vi "Review Fiducials.vi"(7 "Console Log in":refnum<class "Console Log.lvclass">, 8 "error in":errorcluster, 11 "Gluing Procedure in":refnum<class "Gluing Procedure.lvclass">) -> (0 "error out":errorcluster, 1 "Step canceled?":bool, 3 "Gluing Procedure out":refnum<class "Gluing Procedure.lvclass">, 5 "Console Log out":refnum<class "Console Log.lvclass">)   [LabVIEW 2011]
uses:
  Procedure Classes/Gluing Procedure/Gluing Procedure.lvclass
  Application Utilities/Console Log/Console Log.lvclass
  Shared Components/WorkTable Class/Type Definitions/Worktable_Mode.ctl
  Shared Components/Utils/Type Definitions/Fiducial with Source.ctl
  Shared Components/Vec3d Class/Vec3d Class.lvclass
  Procedure Classes/Gluing Procedure/Type Definitions/Review Fuducials.ctl
  Procedure Classes/Gluing Procedure/Type Definitions/Inspect Fuducials.ctl
  Shared Components/Utils/Type Definitions/Part Fiducials.ctl
  Shared Components/Utils/Type Definitions/Fiducial Image.ctl
  Shared Components/Utils/Type Definitions/Physical Image.ctl
  <vilib>/vision/Image Controls.llb/IMAQ Image.ctl
panel:
  in  "idx value":i32
  out "idx_label":string="1/10"
  in  "Previous":bool
  in  "Next":bool
  in  "Path Tab Control":T1(tab)
  out "BBM Slot":i32
  in  "reacquire BBM BL":bool
  in  "reacquire BBM BR":bool
  in  "reacquire BBM TR":bool
  out "BBM TR View":T2(plugin-control)
  out "BBM TL View":T2(plugin-control)
  out "BBM BR View":T2(plugin-control)
  out "BBM BL View":T2(plugin-control)
  in  "reacquire BBM TL":bool
  in  "reacquire HDI TL":bool
  out "HDI BL View":T2(plugin-control)
  out "HDI BR View":T2(plugin-control)
  out "HDI TL View":T2(plugin-control)
  out "HDI TR View":T2(plugin-control)
  in  "reacquire HDI TR":bool
  in  "reacquire HDI BR":bool
  in  "reacquire HDI BL":bool
  out "HDI Slot":i32
  in  "reacquire Stamp BL":bool
  in  "reacquire Stamp BR":bool
  in  "reacquire Stamp TR":bool
  out "Stamp TR View":T2(plugin-control)
  out "Stamp TL View":T2(plugin-control)
  out "Stamp BR View":T2(plugin-control)
  out "Stamp BL View":T2(plugin-control)
  in  "reacquire Stamp TL":bool
  out "Stamp Slot":i32
  in  "reacquire Weight TL":bool
  out "Weight BL View":T2(plugin-control)
  out "Weight BR View":T2(plugin-control)
  out "Weight TL View":T2(plugin-control)
  out "Weight TR View":T2(plugin-control)
  in  "reacquire Weight TR":bool
  in  "reacquire Weight BR":bool
  in  "reacquire Weight BL":bool
  out "Weight Slot":i32
  in  "Cancel Button":bool
  in  "OK Button":bool
  # "This is going to be a monstrous VI.\n\nThis VI needs to display the fiducial images to the user for all HDI, Stamps, Weights, and BBMs.  Users can accept camera's findings or user designate fiducial centers.\n\nHitting okay will write fidicial coords to worktable."
  # "Click on images to correct fiducial positions.\nAll error fiducials must be corrected before continuing."
  # "Pattern Recognition"
  # "Error"
  # "User Defined"
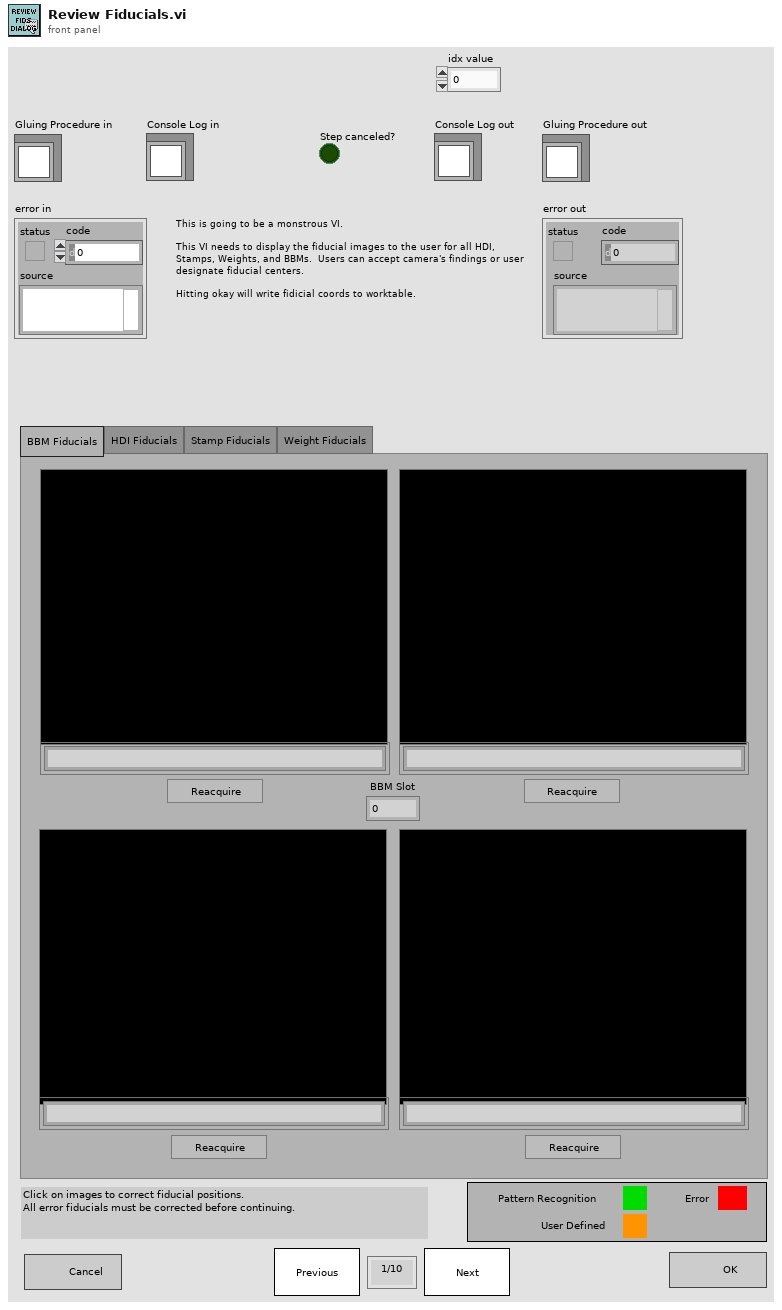
[diagram p1: front panel]
types:
  T1 = enum32{"BBM Fiducials", "HDI Fiducials", "Stamp Fiducials", "Weight Fiducials"}
  T2 = typedef "IMAQ Image.ctl" = refnum<image>
  T3 = cluster{"reacq. HDI":refnum<vi>[], "reacq. Stamp":refnum<vi>[], "reacq. Weight":refnum<vi>[], "reacq. BBM":refnum<vi>[]}
  T4 = typedef "Inspect Fuducials.ctl" = cluster{"Path Fiducials":cluster{"HDI Fiducials":T5, "Stamp Fiducials":T5, "Weight Fiducials":T5, "BBM Fiducials":T5}[], "Has been run?":bool}
  T5 = typedef "Part Fiducials.ctl" = cluster{"Fiducials":T6[], "Chuck":i32, "Slot":i32}
  T6 = typedef "Fiducial Image.ctl" = cluster{"Fiducial Image":T7, "Selected Fiducial":T8, "fiducial name":string}
  T7 = typedef "Physical Image.ctl" = cluster{"Image Position":refnum<class "Vec3d Class.lvclass">, "Image Reference":T2, "Field of View":cluster{"x(mm)":dbl, "y(mm)":dbl}}
  T8 = typedef "Fiducial with Source.ctl" = cluster{"Fiducial Image Coordinate":refnum<class "Vec3d Class.lvclass">, "Fiducial Source":enum16{"Pattern Recognition", "User", "Error", "Default"}}
  T9 = cluster{"HDI Fiducials":T5, "Stamp Fiducials":T5, "Weight Fiducials":T5, "BBM Fiducials":T5}[]
  T10 = typedef "Worktable_Mode.ctl" = enum16{"Encapsulation", "Gluing"}
  T11 = enum16{"None", "glue_resevoir_chuck", "stamp_tool_chuck", "weight_tool_chuck", "hdi_chuck_04"}
  T12 = enum16{"None", "glue_resevoir_chuck", "stamp_tool_chuck", "weight_tool_chuck"}
  T13 = enum16{"Pattern Recognition", "User", "Error", "Default"}
  T14 = typedef "eventvkey.ctl" = enum16{"ASCII", "Enter", "Return", "Shift", "Ctrl", "Alt", "Cmd", "Opt", "Caps", "NumLock", "Clear", "Break", "Up", "Down", "Left", "Right", "Insert", "Delete", "Home", "End", "PageUp", "PageDown", "Escape", "Help", "Pause", "ScrollLock", "F1", "F2", "F3", "F4", "F5", "F6", "F7", "F8", "F9", "F10", "F11", "F12", "F13", "F14", "F15", "F16", "F17", "F18", "F19", "F20", "F21", "F22", "F23", "F24", "Play", "VolumeUp", "VolumeDown", "Mute", "Two Byte Char"}
  T15 = cluster{"HDI Fiducials":T5, "Stamp Fiducials":T5, "Weight Fiducials":T5, "BBM Fiducials":T5}
  T16 = typedef "LVPoint32TypeDef.ctl" = cluster{"Horizontal":i32, "Vertical":i32}
  T17 = typedef "Review Fuducials.ctl" = cluster{"Has been run?":bool}
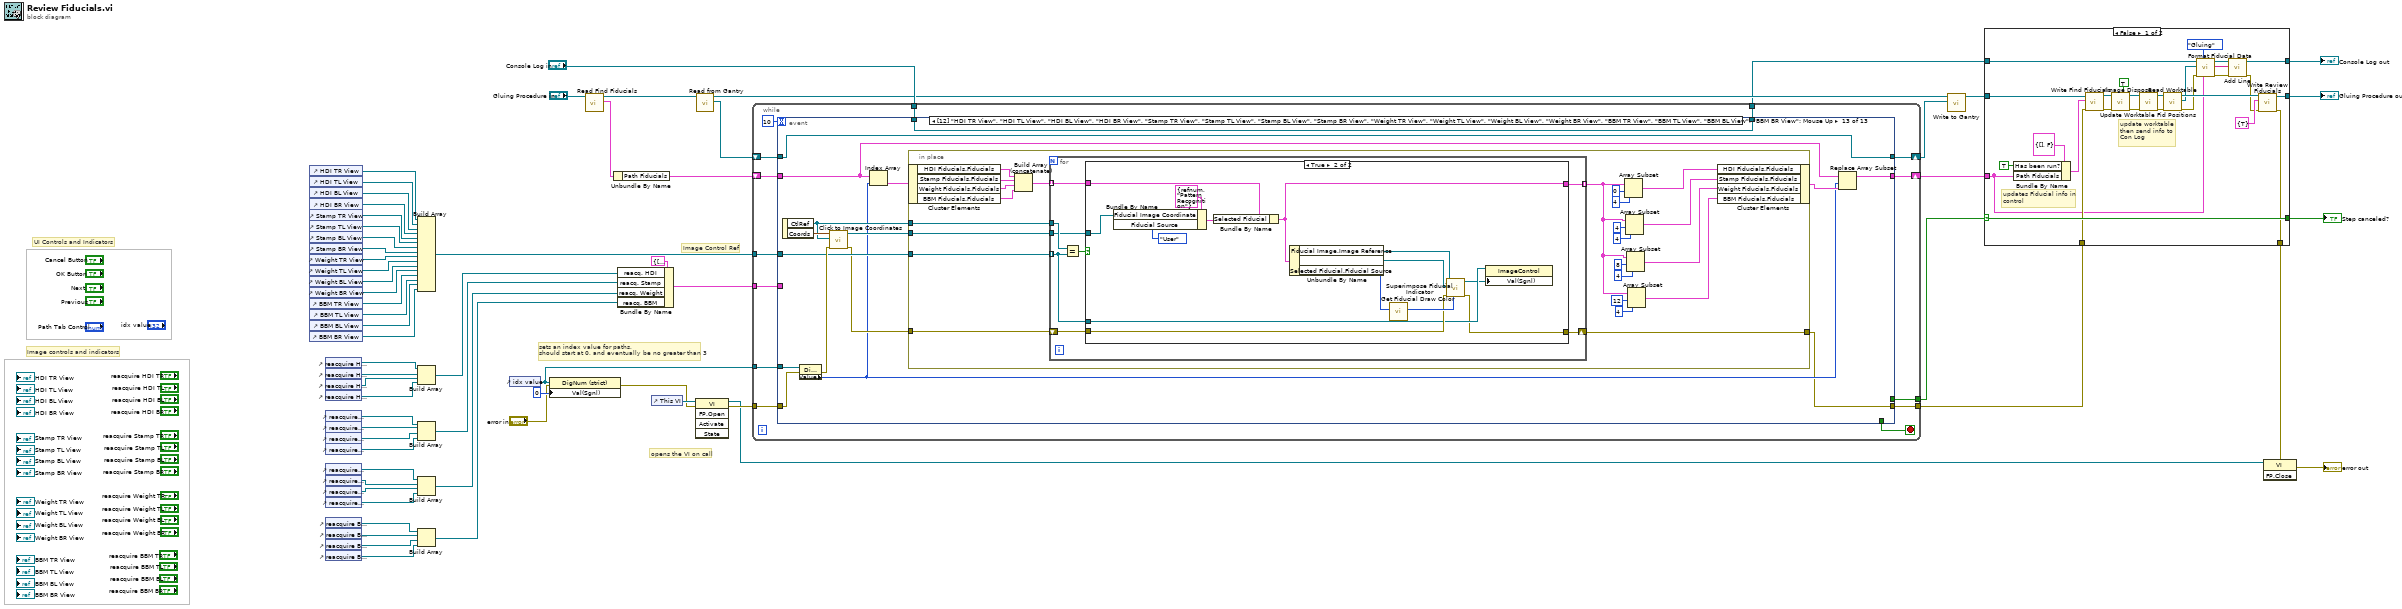
[diagram p0: block diagram]
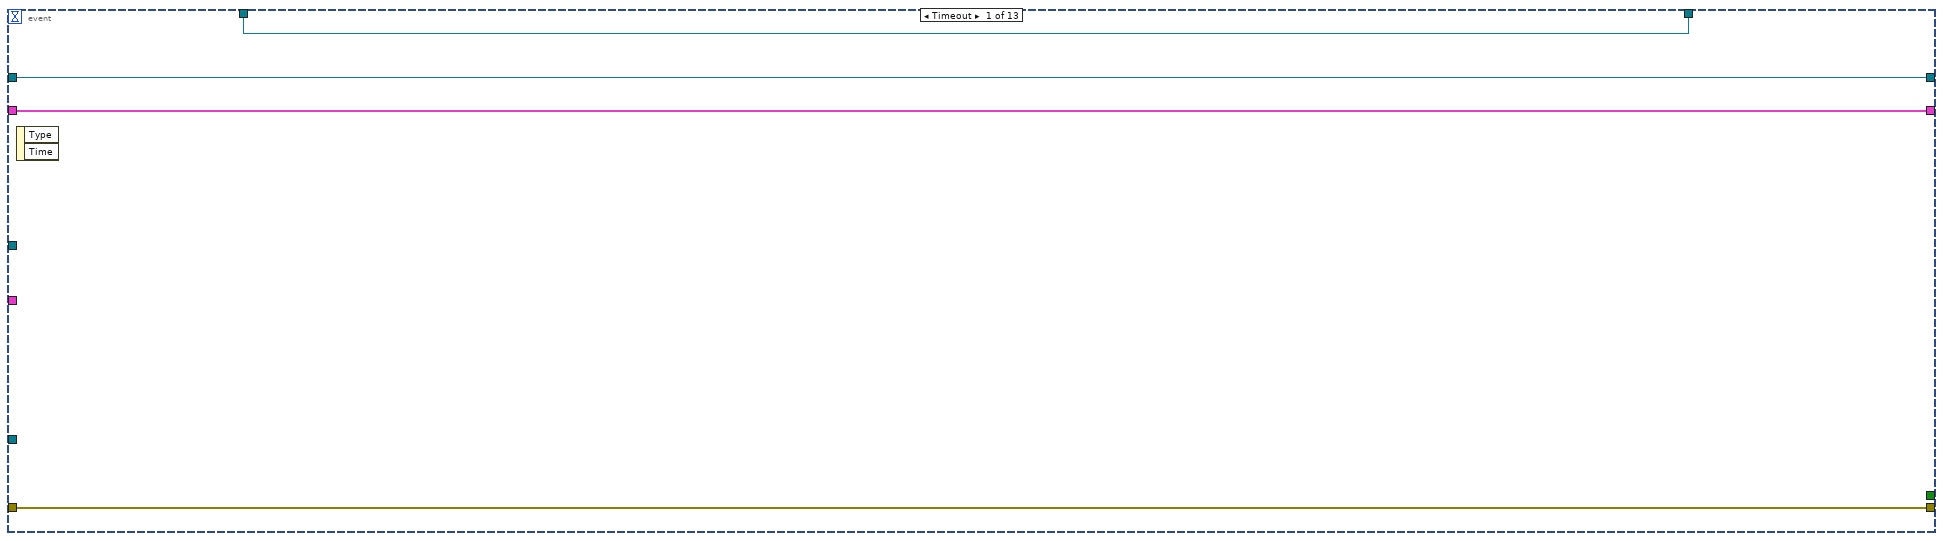
[diagram p3: hidden frame]
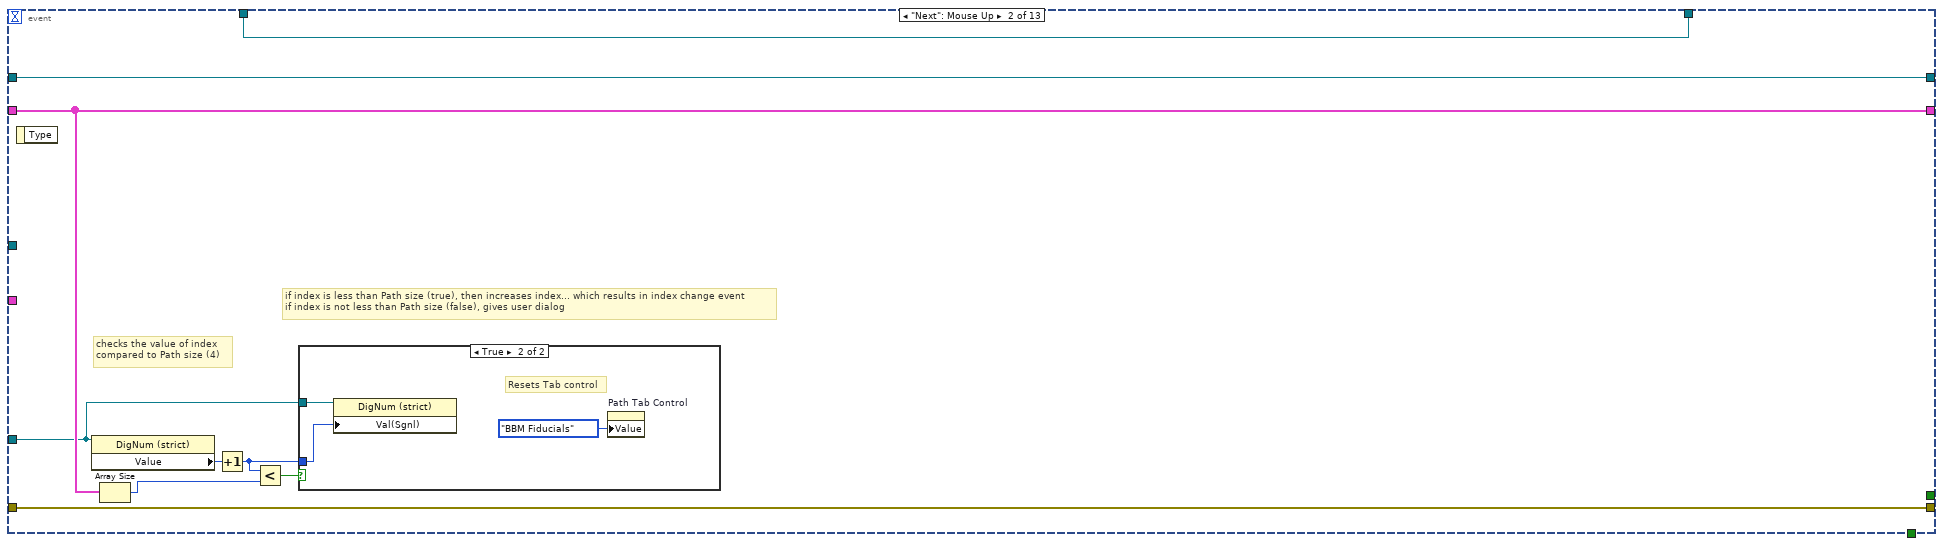
[diagram p4: hidden frame]
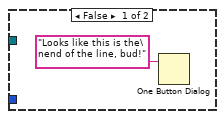
[diagram p5: hidden frame]
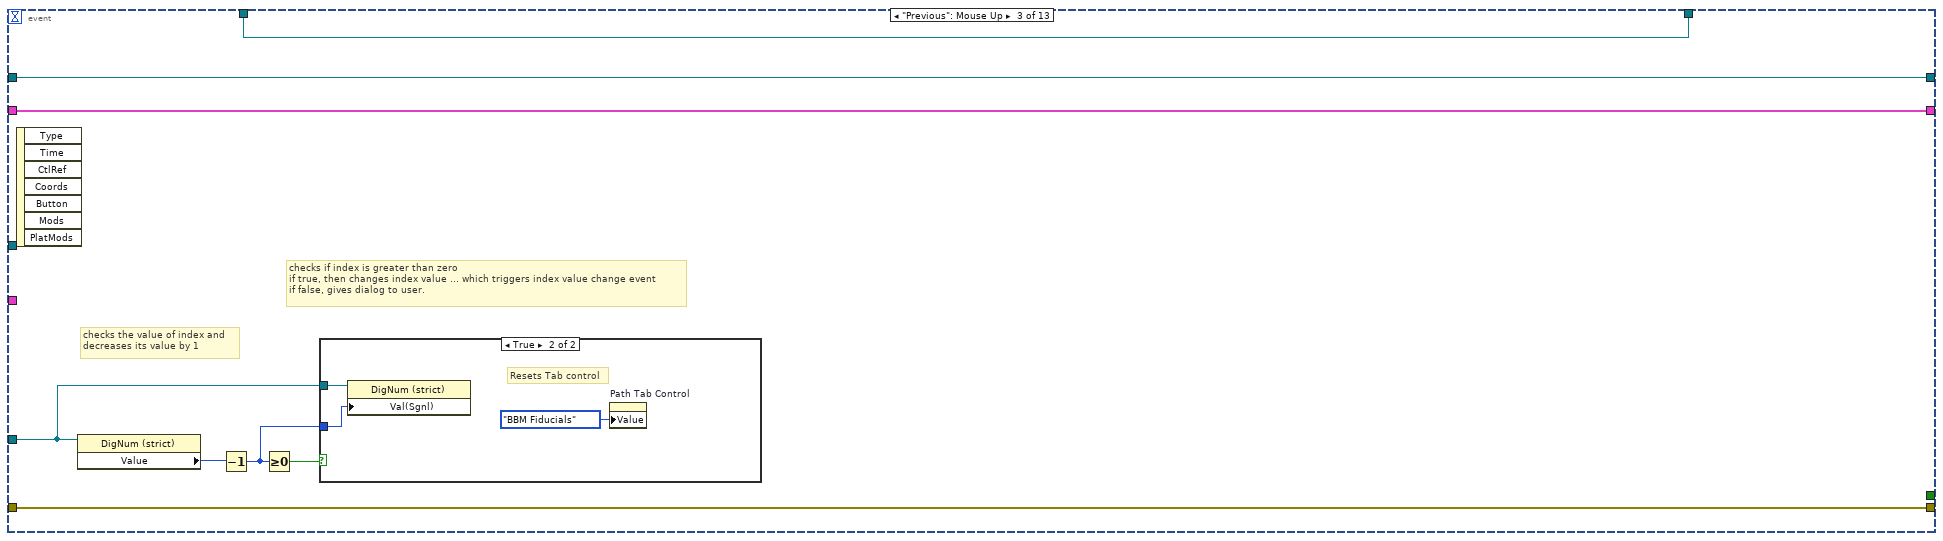
[diagram p6: hidden frame]
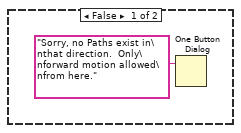
[diagram p7: hidden frame]
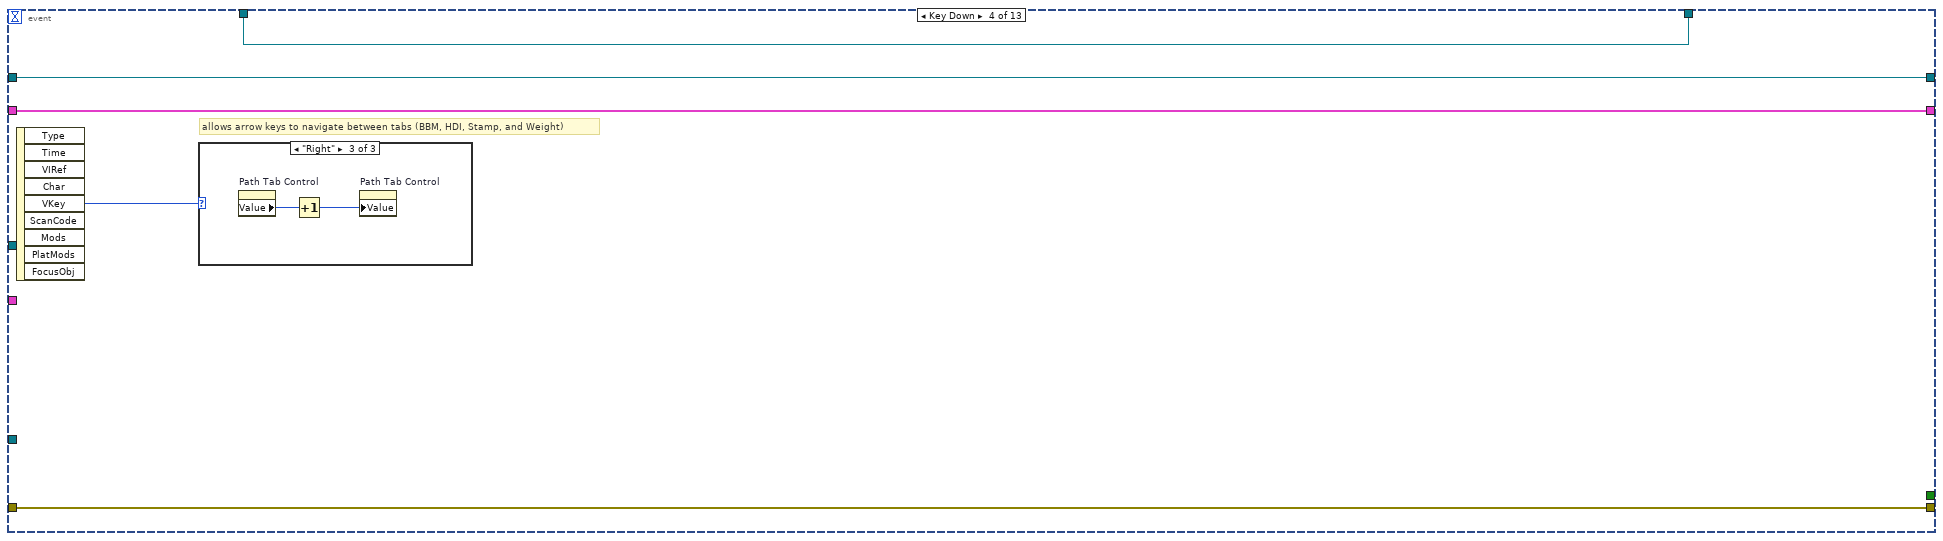
[diagram p8: hidden frame]
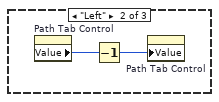
[diagram p10: hidden frame]
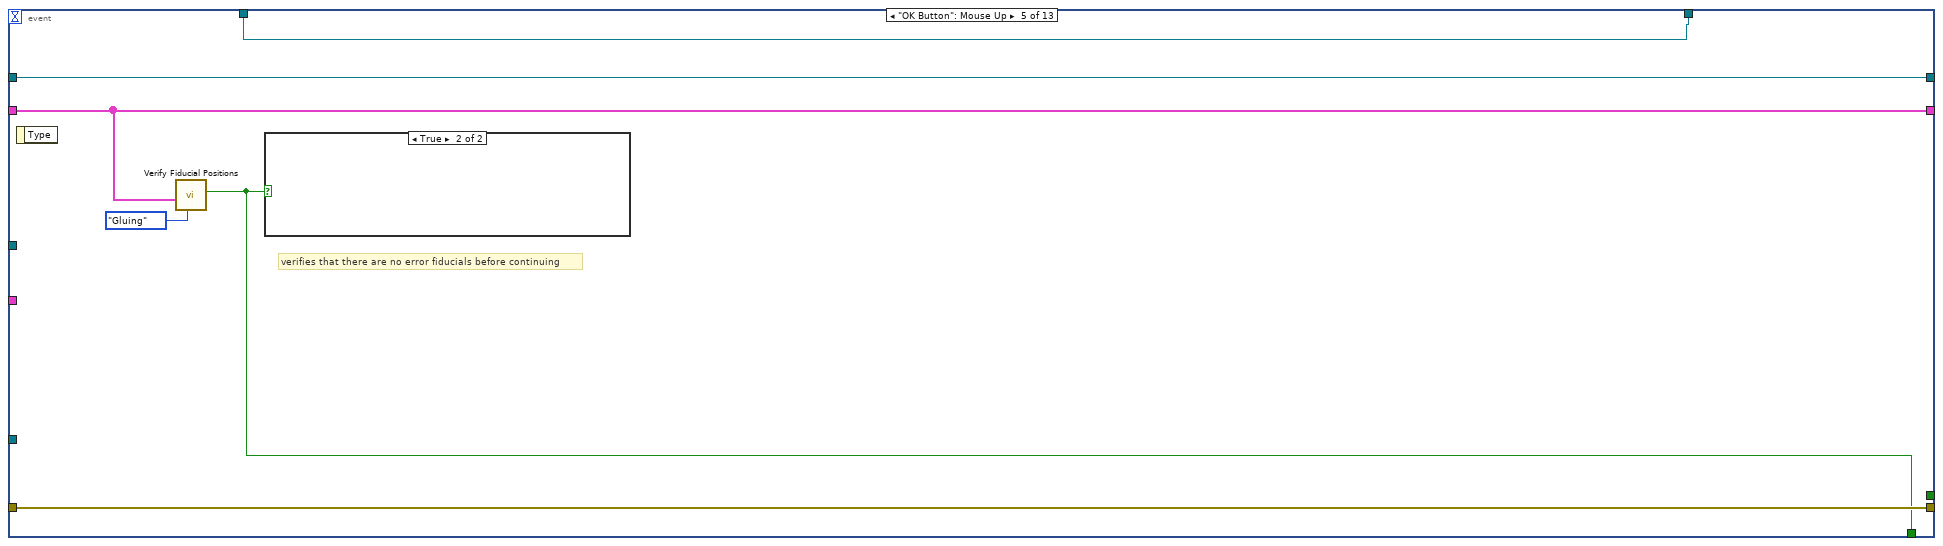
[diagram p11: hidden frame]
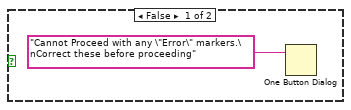
[diagram p12: hidden frame]
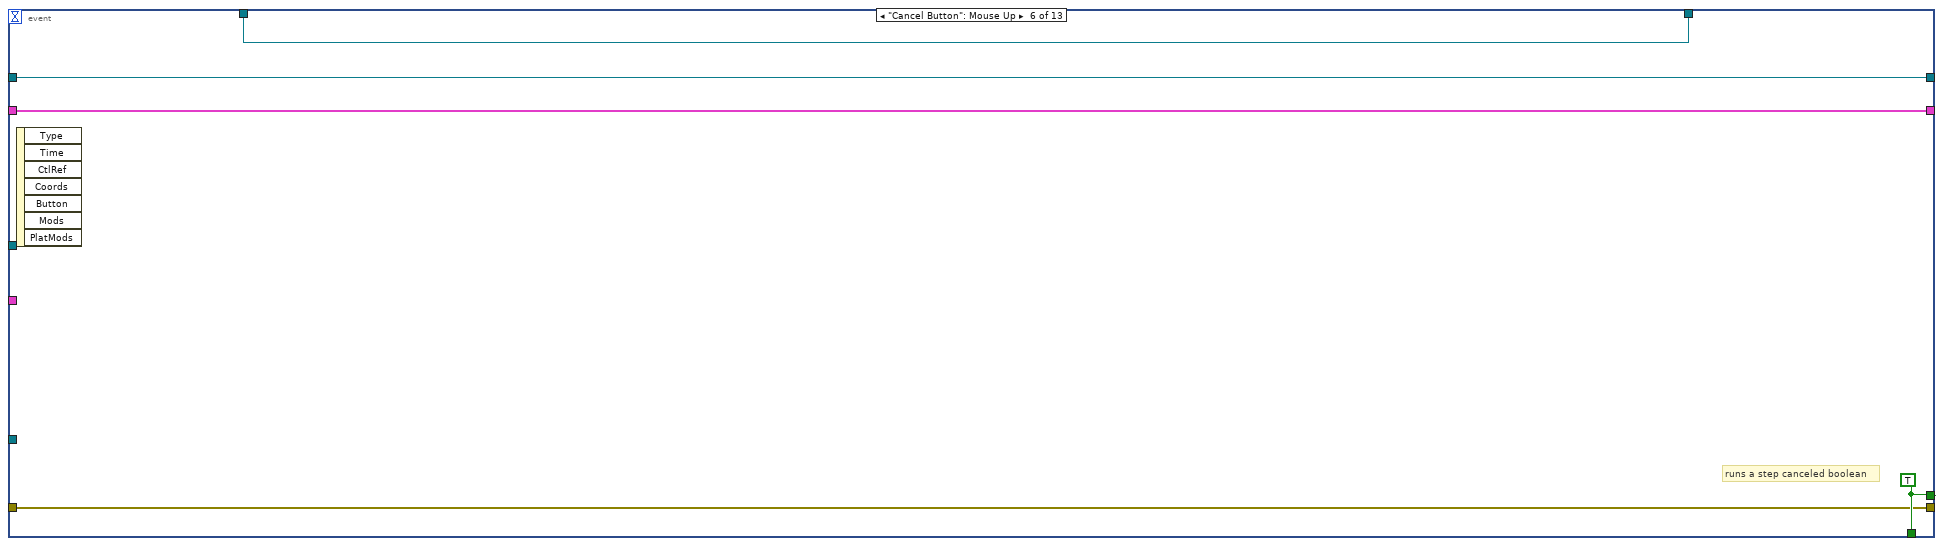
[diagram p13: hidden frame]
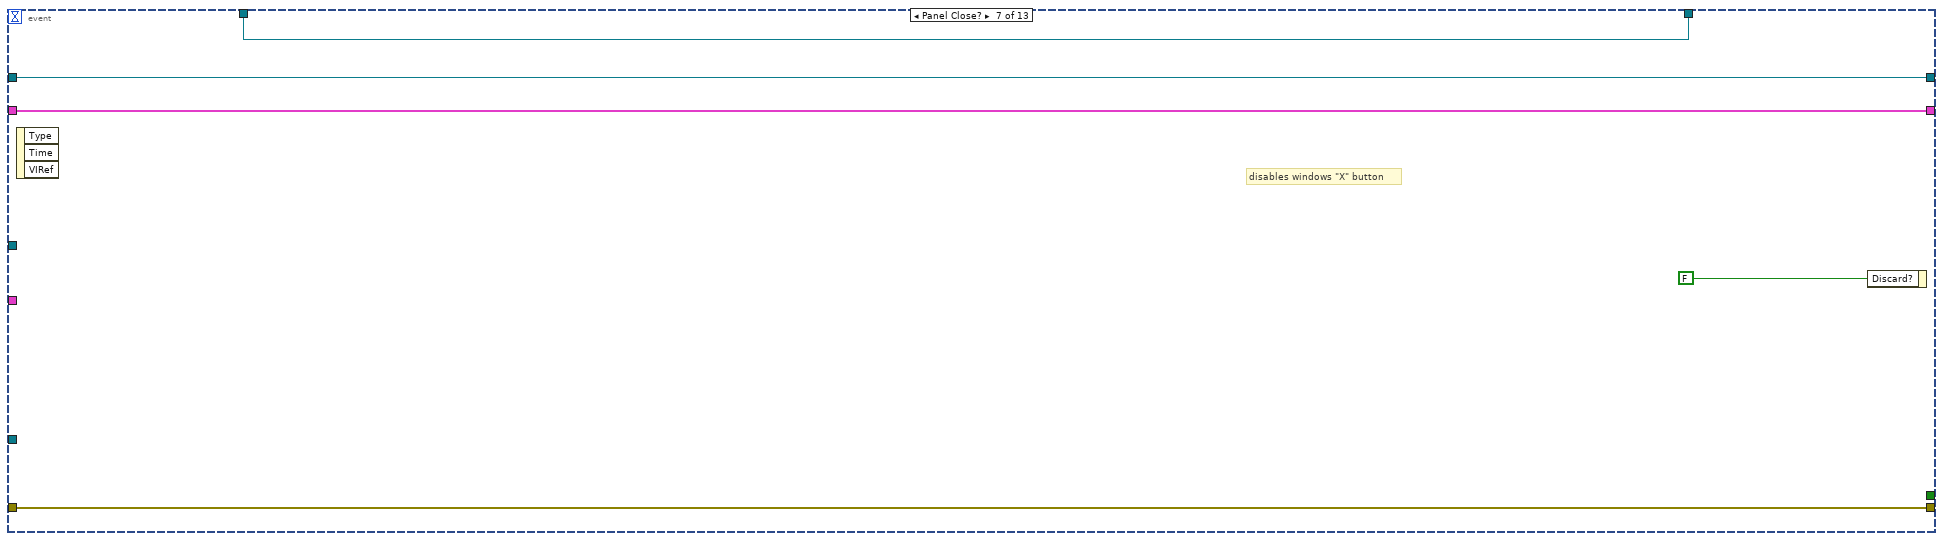
[diagram p14: hidden frame]
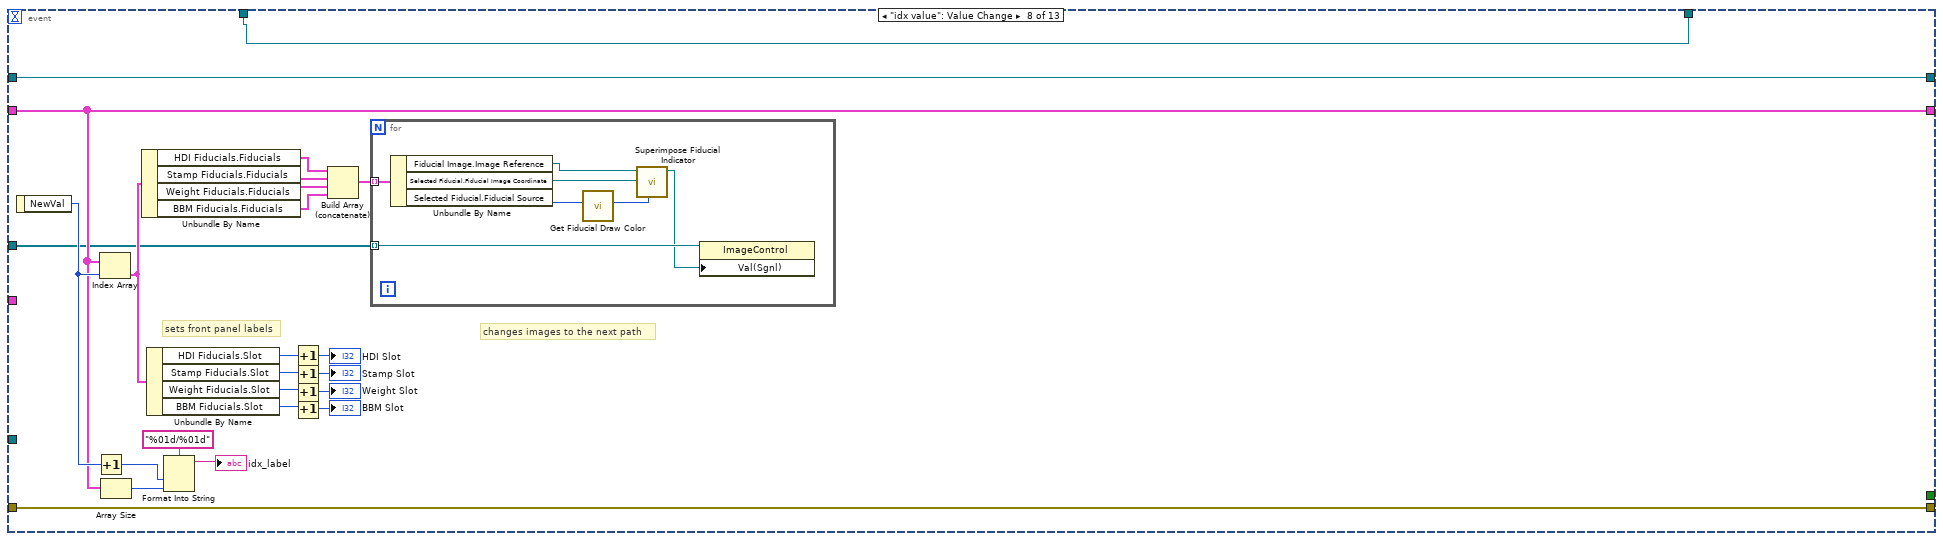
[diagram p15: hidden frame]
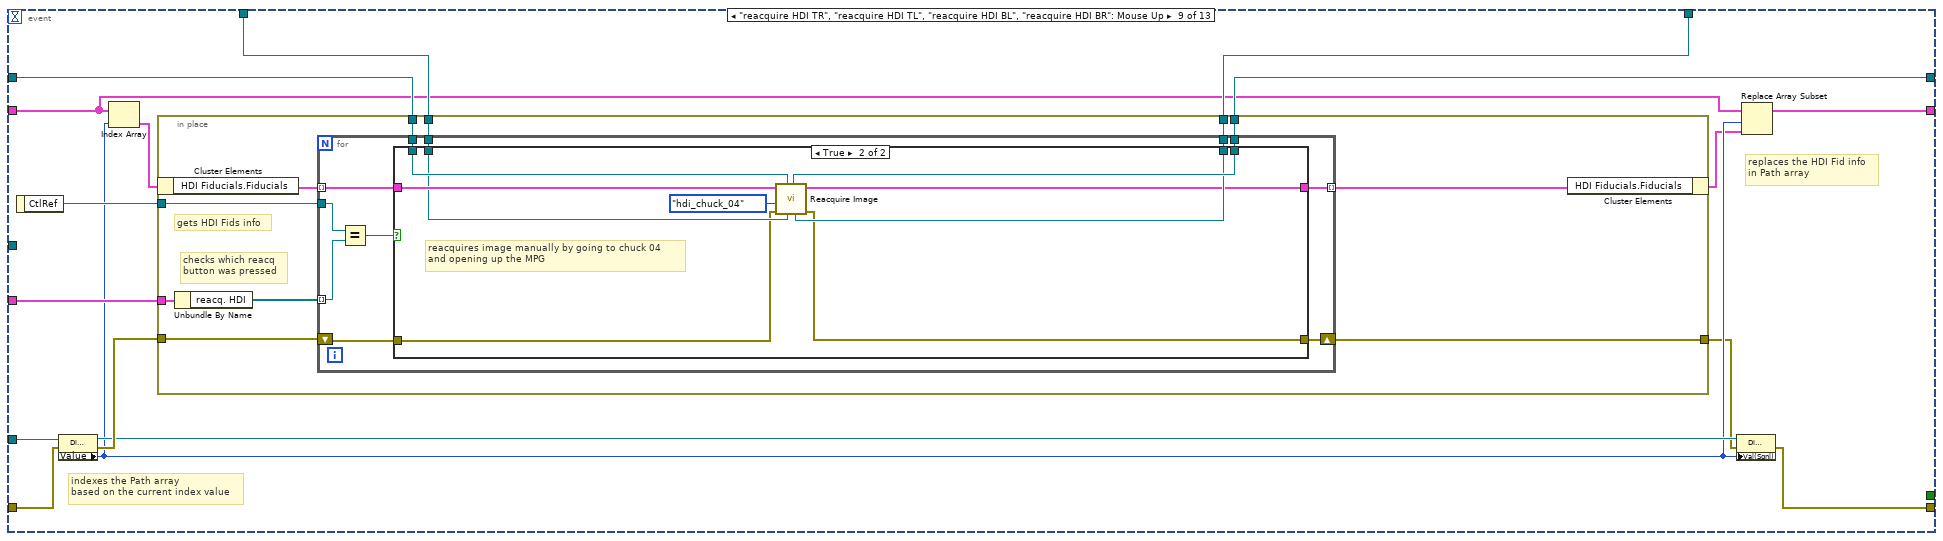
[diagram p16: hidden frame]
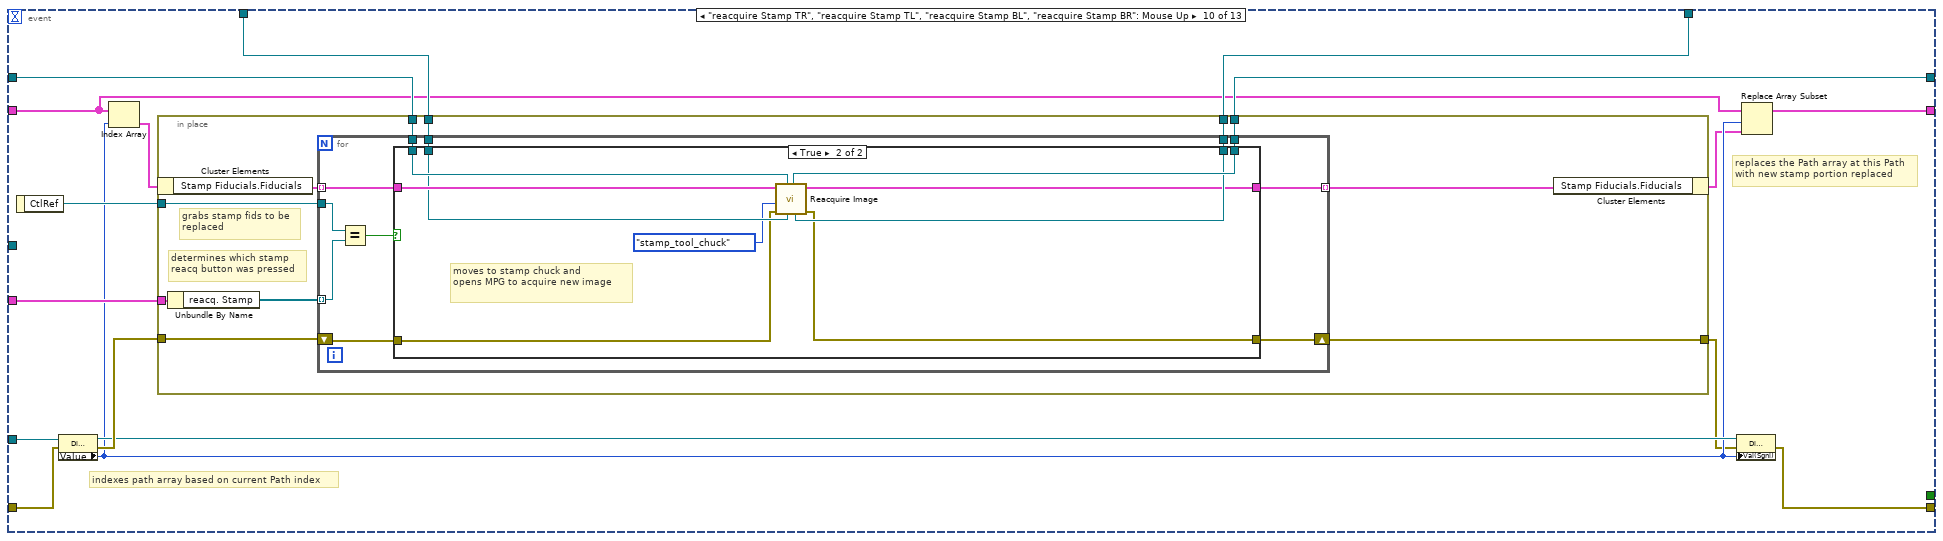
[diagram p18: hidden frame]
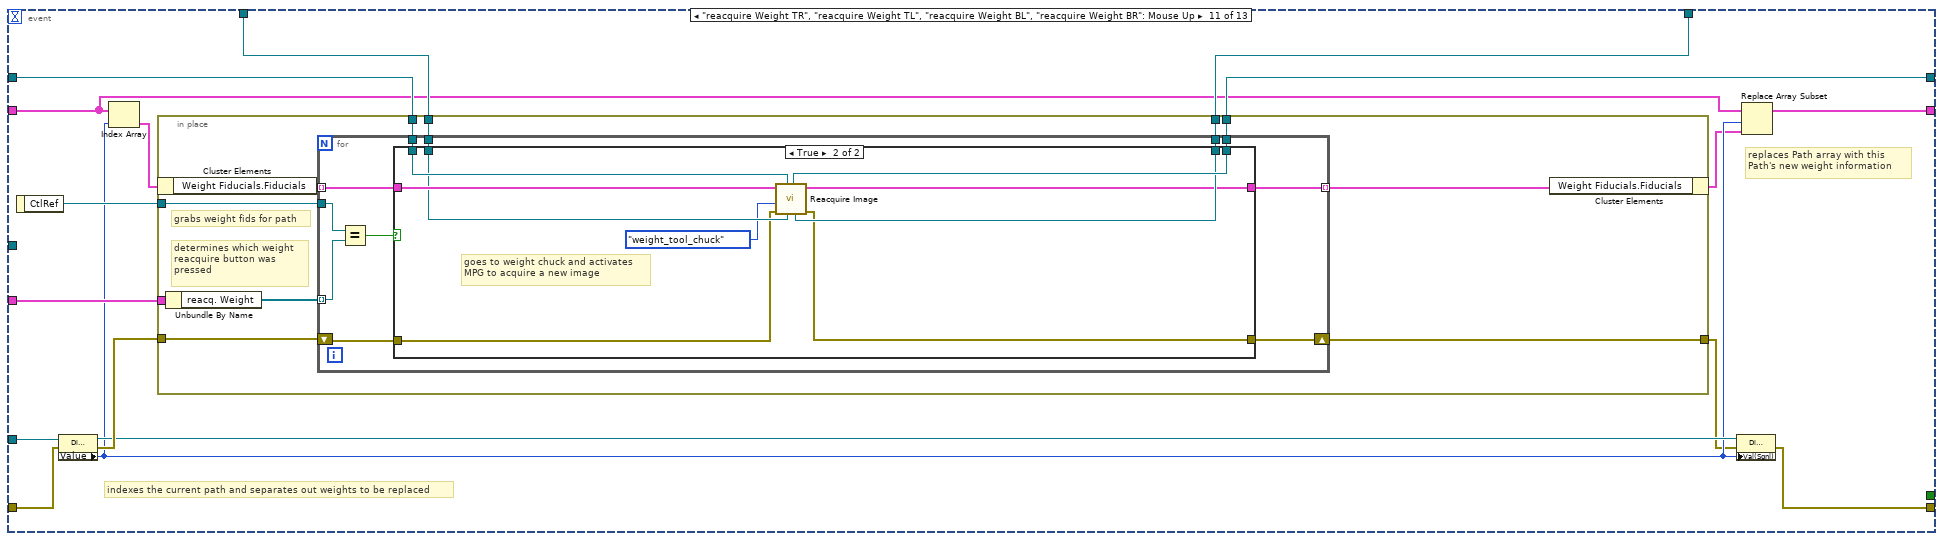
[diagram p20: hidden frame]
diagram:
  # "opens the VI on call"
  # "sets an index value for paths,\nshould start at 0, and eventually be no greater than 3"
  # "Image controls and indicators"
  # "UI Controls and Indicators"
  # "Image Control Ref"
  n1 = control-ref of="HDI TR View"() -> (w54:refnum<vi>)
  n2 = control-ref of="HDI TL View"() -> (w53:refnum<vi>)
  n3 = control-ref of="HDI BL View"() -> (w52:refnum<vi>)
  n4 = control-ref of="HDI BR View"() -> (w51:refnum<vi>)
  n5 = control-ref of="Stamp TR View"() -> (w50:refnum<vi>)
  n6 = control-ref of="Stamp TL View"() -> (w49:refnum<vi>)
  n7 = control-ref of="Stamp BL View"() -> (w48:refnum<vi>)
  n8 = control-ref of="Stamp BR View"() -> (w47:refnum<vi>)
  n9 = control-ref of="Weight TR View"() -> (w46:refnum<vi>)
  n10 = control-ref of="Weight TL View"() -> (w45:refnum<vi>)
  n11 = control-ref of="Weight BL View"() -> (w44:refnum<vi>)
  n12 = control-ref of="Weight BR View"() -> (w43:refnum<vi>)
  n13 = control-ref of="BBM TR View"() -> (w42:refnum<vi>)
  n14 = control-ref of="BBM TL View"() -> (w41:refnum<vi>)
  n15 = control-ref of="BBM BL View"() -> (w40:refnum<vi>)
  n16 = control-ref of="BBM BR View"() -> (w39:refnum<vi>)
  n17 = control-ref of="reacquire HDI TR"() -> (w37:refnum<vi>)
  n18 = control-ref of="reacquire HDI TL"() -> (w36:refnum<vi>)
  n19 = control-ref of="reacquire HDI BL"() -> (w35:refnum<vi>)
  n20 = control-ref of="reacquire HDI BR"() -> (w34:refnum<vi>)
  n21 = control-ref of="reacquire Stamp TR"() -> (w33:refnum<vi>)
  n22 = control-ref of="reacquire Stamp TL"() -> (w32:refnum<vi>)
  n23 = control-ref of="reacquire Stamp BL"() -> (w31:refnum<vi>)
  n24 = control-ref of="reacquire Stamp BR"() -> (w30:refnum<vi>)
  n25 = control-ref of="reacquire Weight TR"() -> (w29:refnum<vi>)
  n26 = control-ref of="reacquire Weight TL"() -> (w28:refnum<vi>)
  n27 = control-ref of="reacquire Weight BL"() -> (w27:refnum<vi>)
  n28 = control-ref of="reacquire Weight BR"() -> (w26:refnum<vi>)
  n29 = control-ref of="reacquire BBM TR"() -> (w25:refnum<vi>)
  n30 = control-ref of="reacquire BBM TL"() -> (w24:refnum<vi>)
  n31 = control-ref of="reacquire BBM BL"() -> (w23:refnum<vi>)
  n32 = control-ref of="reacquire BBM BR"() -> (w22:refnum<vi>)
  n33 = Build Array(w54, w53, w52, w51, w50, w49, w48, w47, w46, w45, w44, w43, w42, w41, w40, w39) -> (w38:refnum<vi>[])
  n34 = Build Array(w37, w36, w35, w34) -> (w20:refnum<vi>[])
  n35 = Build Array(w33, w32, w31, w30) -> (w18:refnum<vi>[])
  n36 = Build Array(w29, w28, w27, w26) -> (w17:refnum<vi>[])
  n37 = Build Array(w25, w24, w23, w22) -> (w16:refnum<vi>[])
  n38 = control-ref of="idx value"() -> (w55:refnum<vi>)
  n39 = property class="DigNum (strict)"(reference=w55, error in="error in", "Val(Sgnl)"=0 ("Value (Signaling)")) -> (error out=w56:errorcluster)  [unwired: 1 out]
  n40 = call "Read Find Fiducials.vi"("Gluing Procedure in"="Gluing Procedure in") -> ("Find Fiducials"=w62:T4, "Gluing Procedure out"=w61:refnum<class "Gluing Procedure.lvclass">)  [unwired: 8 in, 1 out]
  n41 = Unbundle By Name(w62) -> ("Path Fiducials"=w1:T9)
  n42 = Bundle By Name(cluster=T3 {"reacq. HDI"=[], "reacq. Stamp"=[], "reacq. Weight"=[], "reacq. BBM"=[]}, "reacq. HDI"=w20, "reacq. Stamp"=w18, "reacq. Weight"=w17, "reacq. BBM"=w16) -> (w19:T3)
  n43 = control-ref of="This VI"() -> (w64:refnum<vi>)
  n44 = invoke class="VI" method="FP.Open"(reference=w64, error in=w56) -> (reference out=w15:refnum<vi>, error out=w59:errorcluster)  [unwired: 3 in, 3 out]
  n45 = call "Read from Gantry.vi"("Gluing Procedure in"=w61) -> ("Gantry"=w60:refnum<class "Gantry Class.lvclass">, "Gluing Procedure out"=w14:refnum<class "Gluing Procedure.lvclass">)  [unwired: 8 in, 1 out]
  n46 = while {
    tunnel: "Console Log in" -> [w73]
    shift-right: [w75] -> w13
    shift-left: w60 -> [w76]
    shift-right: [w74] -> w9
    shift-left: w1 -> [w77]
    tunnel: [w72] -> w8
    tunnel: w59 -> [w71]
    tunnel: [w70] -> w5
    tunnel: [w68] -> w11
    tunnel: w55 -> [w67]
    tunnel: w38 -> [w66]
    tunnel: w19 -> [w65]
    stop <- w69 stop-if-true
    n47 = event shown="[12] \"HDI TR View\", \"HDI TL View\", \"HDI BL View\", \"HDI BR View\", \"Stamp TR View\", \"Stamp TL View\", \"Stamp BL View\", \"Stamp BR View\", \"Weight TR View\", \"Weight TL View\", \"Weight BL View\", \"Weight BR View\", \"BBM TR View\", \"BBM TL View\", \"BBM BL View\", \"BBM BR View\": Mouse Up" {
      selector: _ -> [_ _ _ _ _ _ _ _ _ _ _ _ _]
      dyn-events: _ -> [_ _ _ _ _ _ _ _ _ _ _ _ _]
      timeout: 10 -> [_ _ _ _ _ _ _ _ _ _ _ _ _]
      tunnel: w77 -> [w81 w89 w102 w110 w120 w127 w131 w154 w170 w222 w274 w326 w383]
      tunnel: w76 -> [w82 w91 w103 w111 w121 w128 w132 w157 w177 w229 w281 w333 w380]
      tunnel: [w82 w91 w103 w111 w121 w128 w132 w157 w176 w228 w280 w332 w380] -> w75
      tunnel: [w81 w89 w102 w110 w120 w127 w131 w154 w167 w219 w271 w323 w381] -> w74
      tunnel: w73 -> [w80 w83 w96 w109 w118 w124 w129 w142 w175 w227 w279 w331 w378]
      tunnel: [w80 w83 w96 w109 w118 w124 w129 w142 w174 w226 w278 w330 w378] -> w72
      tunnel: w71 -> [w79 w90 w101 w108 w122 w125 w130 w156 w180 w232 w284 w336 w391]
      tunnel: [w79 w90 w101 w108 w122 w125 w130 w156 w165 w217 w269 w321 w379] -> w70
      tunnel: [_ _ _ _ w119 w126 _ _ _ _ _ _ _] -> w69
      tunnel: [_ _ _ _ _ w126 _ _ _ _ _ _ _] -> w68
      tunnel: w67 -> [_ w85 w97 _ _ _ _ _ w181 w233 w285 w337 w392]
      tunnel: w66 -> [_ _ _ _ _ _ _ w143 _ _ _ _ w388]
      tunnel: w65 -> [_ _ _ _ _ _ _ _ w173 w225 w277 w329 _]
      event Timeout {
        n48 = event-data() -> ()  [unwired: 1 in, 2 out]
      }
      event "Next": Mouse Up {
        # "if index is less than Path size (true), then increases index... which results in index change event\nif index is not less than Path size (false), gives user dialog"
        # "checks the value of index \ncompared to Path size (4)"
        n49 = event-data() -> ()  [unwired: 1 in, 1 out]
        n50 = property class="DigNum (strict)"(reference=w85) -> ("Value"=w88:i32)  [unwired: 1 in, 2 out]
        n51 = Array Size(array=w89) -> (size(s)=w87:i32)
        n52 = Increment(x=w88) -> (x+1=w84:i32)
        n53 = Less?(x=w84, y=w87) -> (x < y?=w86:bool)
        n54 = case shown="True" w86 {
          tunnel: w85 -> [_ w95]
          tunnel: w84 -> [_ w94]
          frame False {
            n55 = One Button Dialog(message="Looks like this is the\nend of the line, bud!") -> ()  [unwired: 1 in, 1 out]
          }
          frame True {
            # "Resets Tab control"
            n56 = property class="DigNum (strict)"(reference=w95, "Val(Sgnl)"=w94) -> ()  [unwired: 1 in, 2 out]
            n57 = property on="Path Tab Control" class="TabCtl (strict)"("Value"=T1."BBM Fiducials" ("Path Tab Control")) -> ()  [unwired: 2 in, 2 out]
          }
        }
      }
      event "Previous": Mouse Up {
        # "checks if index is greater than zero\nif true, then changes index value ... which triggers index value change event\nif false, gives dialog to user."
        # "checks the value of index and\ndecreases its value by 1"
        n58 = event-data() -> ()  [unwired: 1 in, 7 out]
        n59 = property class="DigNum (strict)"(reference=w97) -> ("Value"=w100:i32)  [unwired: 1 in, 2 out]
        n60 = Decrement(x=w100) -> (x-1=w98:i32)
        n61 = Greater Or Equal To 0?(x=w98) -> (x >= 0?=w99:bool)
        n62 = case shown="True" w99 {
          tunnel: w98 -> [_ w106]
          tunnel: w97 -> [_ w107]
          frame False {
            n63 = One Button Dialog(message="Sorry, no Paths exist in\nthat direction.  Only\nforward motion allowed\nfrom here.") -> ()  [unwired: 1 in, 1 out]
          }
          frame True {
            # "Resets Tab control"
            n64 = property class="DigNum (strict)"(reference=w107, "Val(Sgnl)"=w106) -> ()  [unwired: 1 in, 2 out]
            n65 = property on="Path Tab Control" class="TabCtl (strict)"("Value"=T1."BBM Fiducials" ("Path Tab Control")) -> ()  [unwired: 2 in, 2 out]
          }
        }
      }
      event Key Down {
        # "allows arrow keys to navigate between tabs (BBM, HDI, Stamp, and Weight)"
        n66 = event-data() -> ("VKey"=w112:T14)  [unwired: 1 in, 8 out]
        n67 = case shown="\"Right\"" w112 {
          frame "ASCII", Default {
          }
          frame "Left" {
            n68 = property on="Path Tab Control" class="TabCtl (strict)"() -> ("Value"=w114:T1)  [unwired: 2 in, 2 out]
            n69 = Decrement(x=w114) -> (x-1=w113:T1)
            n70 = property on="Path Tab Control" class="TabCtl (strict)"("Value"=w113) -> ()  [unwired: 2 in, 2 out]
          }
          frame "Right" {
            n71 = property on="Path Tab Control" class="TabCtl (strict)"() -> ("Value"=w116:T1)  [unwired: 2 in, 2 out]
            n72 = Increment(x=w116) -> (x+1=w115:T1)
            n73 = property on="Path Tab Control" class="TabCtl (strict)"("Value"=w115) -> ()  [unwired: 2 in, 2 out]
          }
        }
      }
      event "OK Button": Mouse Up {
        # "verifies that there are no error fiducials before continuing"
        n74 = event-data() -> ()  [unwired: 1 in, 1 out]
        n75 = call "Verify Fiducial Positions.vi"("Procedure Type"=Worktable_Mode."Gluing", "Path Fiducials"=w120) -> ("All Good"=w119:bool)  [unwired: 8 in, 1 out]
        n76 = case shown="True" w119 {
          frame False {
            n77 = One Button Dialog(message="Cannot Proceed with any \"Error\" markers.\nCorrect these before proceeding") -> ()  [unwired: 1 in, 1 out]
          }
          frame True {
          }
        }
      }
      event "Cancel Button": Mouse Up {
        w126 = TRUE
        # "runs a step canceled boolean"
        n78 = event-data() -> ()  [unwired: 1 in, 7 out]
      }
      event Panel Close? {
        # "disables windows \"X\" button"
        n79 = event-data() -> ()  [unwired: 1 in, 3 out]
        n80 = event-data("Discard?"=FALSE) -> ()  [unwired: 1 in, 1 out]
      }
      event "idx value": Value Change {
        # "sets front panel labels"
        # "changes images to the next path"
        n81 = event-data() -> ("NewVal"=w155:i32)  [unwired: 1 in]
        n82 = Increment(x=w155) -> (x+1=w153:i32)
        n83 = Index Array(array=w154, index=w155) -> (element=w149:T15)
        n84 = Array Size(array=w154) -> (size(s)=w152:i32)
        n85 = Unbundle By Name(w149) -> ("HDI Fiducials.Fiducials"=w148:T6[], "Stamp Fiducials.Fiducials"=w147:T6[], "Weight Fiducials.Fiducials"=w146:T6[], "BBM Fiducials.Fiducials"=w145:T6[])
        n86 = Unbundle By Name(w149) -> ("HDI Fiducials.Slot"=w141:i32, "Stamp Fiducials.Slot"=w136:i32, "Weight Fiducials.Slot"=w135:i32, "BBM Fiducials.Slot"=w134:i32)
        n87 = Format Into String(format string="%01d/%01d", w153, w152) -> (resulting string=→"idx_label":string)  [unwired: 2 in, 1 out]
        n88 = Increment(x=w141) -> (x+1=→"HDI Slot":i32)
        n89 = Increment(x=w136) -> (x+1=→"Stamp Slot":i32)
        n90 = Increment(x=w135) -> (x+1=→"Weight Slot":i32)
        n91 = Increment(x=w134) -> (x+1=→"BBM Slot":i32)
        n92 = Build Array (concatenate)(w148, w147, w146, w145) -> (w144:T6[])
        n93 = for {
          tunnel: w144 -> [w164] mode=indexing
          tunnel: w143 -> [w159] mode=indexing
          n94 = Unbundle By Name(w164) -> ("Fiducial Image.Image Reference"=w163:T2, "Selected Fiducial.Fiducial Image Coordinate"=w162:refnum<class "Vec3d Class.lvclass">, "Selected Fiducial.Fiducial Source"=w161:T13)
          n95 = call "Get Fiducial Draw Color.vi"("Fiducial Source"=w161) -> ("Grid Line Color"=w160:u32)  [unwired: 10 in]
          n96 = call "Superimpose Fiducial Indicator.vi"("Marker Color"=w160, "Fiducial Image Coordinates"=w162, "Image In"=w163) -> ("Image Out"=w158:T2)  [unwired: 7 in, 1 out]
          n97 = property class="ImageControl"(reference=w159, "Val(Sgnl)"=w158) -> ()  [unwired: 1 in, 2 out]
        }
      }
      event "reacquire HDI TR", "reacquire HDI TL", "reacquire HDI BL", "reacquire HDI BR": Mouse Up {
        # "replaces the HDI Fid info\nin Path array"
        # "indexes the Path array\nbased on the current index value"
        n98 = event-data() -> ("CtlRef"=w178:refnum<vi>)  [unwired: 1 in]
        n99 = property class="DigNum (strict)"(reference=w181, error in=w180) -> (reference out=w171:refnum<vi>, error out=w172:errorcluster, "Value"=w169:i32)
        n100 = Index Array(array=w170, index=w169) -> (element=w179:T15)
        n101 = in-place {
          in-place-border: w178 -> [w191]
          in-place-border: w177 -> [w190]
          in-place-border: [w189] -> w176
          in-place-border: w175 -> [w188]
          in-place-border: [w187] -> w174
          in-place-border: w173 -> [w185]
          in-place-border: w172 -> [w183]
          in-place-border: [w182] -> w166
          # "checks which reacq\nbutton was pressed"
          # "gets HDI Fids info"
          n102 = in-place-cluster #1(w179) -> ("HDI Fiducials.Fiducials"=w192:T6[])
          n103 = Unbundle By Name(w185) -> ("reacq. HDI"=w184:refnum<vi>[])
          n104 = for {
            tunnel: w192 -> [w199] mode=indexing
            tunnel: w191 -> [w203]
            tunnel: w184 -> [w202] mode=indexing
            tunnel: w190 -> [w200]
            tunnel: [w198] -> w189
            tunnel: w188 -> [w197]
            tunnel: [w196] -> w187
            tunnel: [w195] -> w186 mode=indexing
            shift-right: [w193] -> w182
            shift-left: w183 -> [w194]
            n105 = Equal?(x=w203, y=w202) -> (x = y?=w201:bool)
            n106 = case shown="True" w201 {
              tunnel: w200 -> [w206 w215]
              tunnel: w199 -> [w207 w216]
              tunnel: [w206 w214] -> w198
              tunnel: w197 -> [w205 w213]
              tunnel: [w205 w212] -> w196
              tunnel: [w207 w211] -> w195
              tunnel: w194 -> [w204 w210]
              tunnel: [w204 w209] -> w193
              frame False {
                # "False means this was not the selected reacquire button"
              }
              frame True {
                # "reacquires image manually by going to chuck 04\nand opening up the MPG"
                n107 = call "Reacquire Image.vi"("Console Log in"=w213, "Gantry in"=w215, "error in"=w210, "Tool Chuck?"=T11."hdi_chuck_04", "Fiducial Image In"=w216) -> ("error out"=w209:errorcluster, "Fiducial Image Out"=w211:T6, "Console Log out"=w212:refnum<class "Console Log.lvclass">, "Gantry out"=w214:refnum<class "Gantry Class.lvclass">)  [unwired: 3 in]
              }
            }
          }
          n108 = in-place-cluster #1("HDI Fiducials.Fiducials"=w186) -> (w168:T15)
        }
        n109 = property class="DigNum (strict)"(reference=w171, error in=w166, "Val(Sgnl)"=w169) -> (error out=w165:errorcluster)  [unwired: 1 out]
        n110 = Replace Array Subset(array=w170, new element=w168, index=w169) -> (w167:T9)
      }
      event "reacquire Stamp TR", "reacquire Stamp TL", "reacquire Stamp BL", "reacquire Stamp BR": Mouse Up {
        # "replaces the Path array at this Path\nwith new stamp portion replaced"
        # "indexes path array based on current Path index"
        n111 = event-data() -> ("CtlRef"=w230:refnum<vi>)  [unwired: 1 in]
        n112 = property class="DigNum (strict)"(reference=w233, error in=w232) -> (reference out=w223:refnum<vi>, error out=w224:errorcluster, "Value"=w221:i32)
        n113 = Index Array(array=w222, index=w221) -> (element=w231:T15)
        n114 = in-place {
          in-place-border: w230 -> [w243]
          in-place-border: w229 -> [w242]
          in-place-border: [w241] -> w228
          in-place-border: w227 -> [w240]
          in-place-border: [w239] -> w226
          in-place-border: w225 -> [w237]
          in-place-border: w224 -> [w235]
          in-place-border: [w234] -> w218
          # "grabs stamp fids to be\nreplaced"
          # "determines which stamp\nreacq button was pressed"
          n115 = in-place-cluster #2(w231) -> ("Stamp Fiducials.Fiducials"=w244:T6[])
          n116 = Unbundle By Name(w237) -> ("reacq. Stamp"=w236:refnum<vi>[])
          n117 = for {
            tunnel: w244 -> [w251] mode=indexing
            tunnel: w243 -> [w255]
            tunnel: w236 -> [w254] mode=indexing
            tunnel: w242 -> [w252]
            tunnel: [w250] -> w241
            tunnel: w240 -> [w249]
            tunnel: [w248] -> w239
            tunnel: [w247] -> w238 mode=indexing
            shift-right: [w245] -> w234
            shift-left: w235 -> [w246]
            n118 = Equal?(x=w255, y=w254) -> (x = y?=w253:bool)
            n119 = case shown="True" w253 {
              tunnel: w252 -> [w258 w267]
              tunnel: w251 -> [w259 w268]
              tunnel: [w258 w266] -> w250
              tunnel: w249 -> [w257 w265]
              tunnel: [w257 w264] -> w248
              tunnel: [w259 w263] -> w247
              tunnel: w246 -> [w256 w262]
              tunnel: [w256 w261] -> w245
              frame False {
                # "False means this was not the stamp reacquire button pressed"
              }
              frame True {
                # "moves to stamp chuck and\nopens MPG to acquire new image"
                n120 = call "Reacquire Image.vi"("Console Log in"=w265, "Gantry in"=w267, "error in"=w262, "Tool Chuck?"=T12."stamp_tool_chuck", "Fiducial Image In"=w268) -> ("error out"=w261:errorcluster, "Fiducial Image Out"=w263:T6, "Console Log out"=w264:refnum<class "Console Log.lvclass">, "Gantry out"=w266:refnum<class "Gantry Class.lvclass">)  [unwired: 3 in]
              }
            }
          }
          n121 = in-place-cluster #2("Stamp Fiducials.Fiducials"=w238) -> (w220:T15)
        }
        n122 = property class="DigNum (strict)"(reference=w223, error in=w218, "Val(Sgnl)"=w221) -> (error out=w217:errorcluster)  [unwired: 1 out]
        n123 = Replace Array Subset(array=w222, new element=w220, index=w221) -> (w219:T9)
      }
      event "reacquire Weight TR", "reacquire Weight TL", "reacquire Weight BL", "reacquire Weight BR": Mouse Up {
        # "indexes the current path and separates out weights to be replaced"
        # "replaces Path array with this\nPath's new weight information"
        n124 = event-data() -> ("CtlRef"=w282:refnum<vi>)  [unwired: 1 in]
        n125 = property class="DigNum (strict)"(reference=w285, error in=w284) -> (reference out=w275:refnum<vi>, error out=w276:errorcluster, "Value"=w273:i32)
        n126 = Index Array(array=w274, index=w273) -> (element=w283:T15)
        n127 = in-place {
          in-place-border: w282 -> [w295]
          in-place-border: w281 -> [w294]
          in-place-border: [w293] -> w280
          in-place-border: w279 -> [w292]
          in-place-border: [w291] -> w278
          in-place-border: w277 -> [w289]
          in-place-border: w276 -> [w287]
          in-place-border: [w286] -> w270
          # "determines which weight\nreacquire button was \npressed"
          # "grabs weight fids for path"
          n128 = in-place-cluster #3(w283) -> ("Weight Fiducials.Fiducials"=w296:T6[])
          n129 = Unbundle By Name(w289) -> ("reacq. Weight"=w288:refnum<vi>[])
          n130 = for {
            tunnel: w296 -> [w303] mode=indexing
            tunnel: w295 -> [w307]
            tunnel: w288 -> [w306] mode=indexing
            tunnel: w294 -> [w304]
            tunnel: [w302] -> w293
            tunnel: w292 -> [w301]
            tunnel: [w300] -> w291
            tunnel: [w299] -> w290 mode=indexing
            shift-right: [w297] -> w286
            shift-left: w287 -> [w298]
            n131 = Equal?(x=w307, y=w306) -> (x = y?=w305:bool)
            n132 = case shown="True" w305 {
              tunnel: w304 -> [w310 w319]
              tunnel: w303 -> [w311 w320]
              tunnel: [w310 w318] -> w302
              tunnel: w301 -> [w309 w317]
              tunnel: [w309 w316] -> w300
              tunnel: [w311 w315] -> w299
              tunnel: w298 -> [w308 w314]
              tunnel: [w308 w313] -> w297
              frame False {
                # "False means this is not the reacquire button that was pressed"
              }
              frame True {
                # "goes to weight chuck and activates\nMPG to acquire a new image"
                n133 = call "Reacquire Image.vi"("Console Log in"=w317, "Gantry in"=w319, "error in"=w314, "Tool Chuck?"=T12."weight_tool_chuck", "Fiducial Image In"=w320) -> ("error out"=w313:errorcluster, "Fiducial Image Out"=w315:T6, "Console Log out"=w316:refnum<class "Console Log.lvclass">, "Gantry out"=w318:refnum<class "Gantry Class.lvclass">)  [unwired: 3 in]
              }
            }
          }
          n134 = in-place-cluster #3("Weight Fiducials.Fiducials"=w290) -> (w272:T15)
        }
        n135 = property class="DigNum (strict)"(reference=w275, error in=w270, "Val(Sgnl)"=w273) -> (error out=w269:errorcluster)  [unwired: 1 out]
        n136 = Replace Array Subset(array=w274, new element=w272, index=w273) -> (w271:T9)
      }
      event "reacquire BBM TR", "reacquire BBM TL", "reacquire BBM BL", "reacquire BBM BR": Mouse Up {
        # "indexes current path, and\nreplaces the BBM info in \ncurrent path"
        # "indexes the current path and separates out BBM info"
        n137 = event-data() -> ("CtlRef"=w334:refnum<vi>)  [unwired: 1 in]
        n138 = property class="DigNum (strict)"(reference=w337, error in=w336) -> (reference out=w327:refnum<vi>, error out=w328:errorcluster, "Value"=w325:i32)
        n139 = Index Array(array=w326, index=w325) -> (element=w335:T15)
        n140 = in-place {
          in-place-border: w334 -> [w349]
          in-place-border: w333 -> [w348]
          in-place-border: [w347] -> w332
          in-place-border: w331 -> [w346]
          in-place-border: [w345] -> w330
          in-place-border: w329 -> [w343]
          in-place-border: w328 -> [w341]
          in-place-border: [w340] -> w322
          # "determines which BBM\nreacq. was pressed"
          # "grabs BBM info"
          n141 = in-place-cluster #4(w335) -> ("BBM Fiducials.Fiducials"=w350:T6[], "BBM Fiducials.Chuck"=w339:i32)
          n142 = Unbundle By Name(w343) -> ("reacq. BBM"=w342:refnum<vi>[])
          n143 = for {
            tunnel: w350 -> [w359] mode=indexing
            tunnel: w349 -> [w363]
            tunnel: w342 -> [w362] mode=indexing
            tunnel: w348 -> [w360]
            tunnel: [w358] -> w347
            tunnel: w346 -> [w357]
            tunnel: [w356] -> w345
            tunnel: [w355] -> w344 mode=indexing
            shift-right: [w353] -> w340
            shift-left: w341 -> [w354]
            shift-right: [w351] -> w338
            shift-left: w339 -> [w352]
            n144 = Equal?(x=w363, y=w362) -> (x = y?=w361:bool)
            n145 = case shown="True" w361 {
              tunnel: w360 -> [w367 w376]
              tunnel: w359 -> [w368 w377]
              tunnel: [w367 w375] -> w358
              tunnel: w357 -> [w366 w374]
              tunnel: [w366 w373] -> w356
              tunnel: [w368 w372] -> w355
              tunnel: w354 -> [w365 w371]
              tunnel: [w365 w370] -> w353
              tunnel: w352 -> [w364 w369]
              tunnel: [w364 w369] -> w351
              frame False {
              }
              frame True {
                # "goes to the BBM chuck and activates MPG"
                n146 = call "Reacquire Image.vi"("Console Log in"=w374, "Gantry in"=w376, "error in"=w371, "Chuck"=w369, "Fiducial Image In"=w377) -> ("error out"=w370:errorcluster, "Fiducial Image Out"=w372:T6, "Console Log out"=w373:refnum<class "Console Log.lvclass">, "Gantry out"=w375:refnum<class "Gantry Class.lvclass">)  [unwired: 3 in]
              }
            }
          }
          n147 = in-place-cluster #4("BBM Fiducials.Fiducials"=w344, "BBM Fiducials.Chuck"=w338) -> (w324:T15)
        }
        n148 = property class="DigNum (strict)"(reference=w327, error in=w322, "Val(Sgnl)"=w325) -> (error out=w321:errorcluster)  [unwired: 1 out]
        n149 = Replace Array Subset(array=w326, new element=w324, index=w325) -> (w323:T9)
      }
      event "HDI TR View", "HDI TL View", "HDI BL View", "HDI BR View", "Stamp TR View", "Stamp TL View", "Stamp BL View", "Stamp BR View", "Weight TR View", "Weight TL View", "Weight BL View", "Weight BR View", "BBM TR View", "BBM TL View", "BBM BL View", "BBM BR View": Mouse Up {
        n150 = event-data() -> ("CtlRef"=w385:refnum<vi>, "Coords"=w393:T16)  [unwired: 1 in]
        n151 = property class="DigNum (strict)"(reference=w392, error in=w391) -> (error out=w390:errorcluster, "Value"=w382:i32)  [unwired: 1 out]
        n152 = call "Click to Image Coordinates.vi"("error in"=w390, "Display Reference"=w385, "Coords"=w393) -> ("error out"=w386:errorcluster, "Image Coordinates"=w387:refnum<class "Vec3d Class.lvclass">)  [unwired: 7 in]
        n153 = Index Array(array=w383, index=w382) -> (element=w389:T15)
        n154 = in-place {
          in-place-border: w388 -> [w411]
          in-place-border: w387 -> [w410]
          in-place-border: w386 -> [w409]
          in-place-border: w385 -> [w408]
          in-place-border: [w394] -> w379
          n155 = in-place-cluster #5(w389) -> ("HDI Fiducials.Fiducials"=w416:T6[], "Stamp Fiducials.Fiducials"=w415:T6[], "Weight Fiducials.Fiducials"=w414:T6[], "BBM Fiducials.Fiducials"=w413:T6[])
          n156 = Build Array (concatenate)(w416, w415, w414, w413) -> (w412:T6[])
          n157 = for {
            tunnel: w412 -> [w422] mode=indexing
            tunnel: w411 -> [w419] mode=indexing
            tunnel: w410 -> [w421]
            tunnel: w408 -> [w424]
            shift-right: [w418] -> w394
            shift-left: w409 -> [w420]
            tunnel: [w417] -> w398 mode=indexing
            n158 = Equal?(x=w424, y=w419) -> (x = y?=w423:bool)
            n159 = case shown="True" w423 {
              tunnel: w422 -> [w426 w440]
              tunnel: w421 -> [_ w438]
              tunnel: w420 -> [w425 w431]
              tunnel: w419 -> [_ w430]
              tunnel: [w425 w428] -> w418
              tunnel: [w426 w427] -> w417
              frame False {
              }
              frame True {
                n160 = Bundle By Name(cluster=T8 {"Fiducial Image Coordinate"=refnum, "Fiducial Source"=enum."Pattern Recognition"} ("Fiducial with Source"), "Fiducial Image Coordinate"=w438, "Fiducial Source"=T13."User") -> (w436:T8)
                n161 = Bundle By Name(cluster=w440, "Selected Fiducial"=w436) -> (w427:T6)
                n162 = Unbundle By Name(w427) -> ("Fiducial Image.Image Reference"=w432:T2, "Selected Fiducial.Fiducial Image Coordinate"=w433:refnum<class "Vec3d Class.lvclass">, "Selected Fiducial.Fiducial Source"=w435:T13)
                n163 = call "Get Fiducial Draw Color.vi"("Fiducial Source"=w435) -> ("Grid Line Color"=w434:u32)  [unwired: 10 in]
                n164 = call "Superimpose Fiducial Indicator.vi"("Marker Color"=w434, "error in"=w431, "Fiducial Image Coordinates"=w433, "Image In"=w432) -> ("error out"=w428:errorcluster, "Image Out"=w429:T2)  [unwired: 6 in]
                n165 = property class="ImageControl"(reference=w430, "Val(Sgnl)"=w429) -> ()  [unwired: 1 in, 2 out]
              }
            }
          }
          n166 = Array Subset(array=w398, index=0, length=4) -> (w405:T6[])
          n167 = Array Subset(array=w398, index=4, length=4) -> (w397:T6[])
          n168 = Array Subset(array=w398, index=8, length=4) -> (w396:T6[])
          n169 = Array Subset(array=w398, index=12, length=4) -> (w395:T6[])
          n170 = in-place-cluster #5("HDI Fiducials.Fiducials"=w405, "Stamp Fiducials.Fiducials"=w397, "Weight Fiducials.Fiducials"=w396, "BBM Fiducials.Fiducials"=w395) -> (w384:T15)
        }
        n171 = Replace Array Subset(array=w383, new element=w384, index=w382) -> (w381:T9)
      }
    }
  }
  n172 = call "Write to Gantry.vi"("Gantry"=w13, "Gluing Procedure in"=w14) -> ("Gluing Procedure out"=w12:refnum<class "Gluing Procedure.lvclass">)  [unwired: 8 in, 1 out]
  n173 = case shown="False" w11 {
    selector: w11 -> [w467 w469]
    tunnel: w12 -> [w466 w470]
    tunnel: [w467 w469] -> w10
    tunnel: w9 -> [w443 _]
    tunnel: w8 -> [w441 w471]
    tunnel: [w450 w471] -> w7
    tunnel: [w460 w470] -> w6
    tunnel: w5 -> [w459 w468]
    tunnel: [w458 w468] -> w4
    frame False {
      # "update worktable\nthen send info to \nCon Log"
      # "updates Fiducial info in\ncontrol"
      n174 = Bundle By Name(cluster=T4 {"Path Fiducials"=[], "Has been run?"=FALSE} ("Find Fiducials"), "Has been run?"=TRUE, "Path Fiducials"=w443) -> (w463:T4)
      n175 = call "Write Find Fiducials.vi"("error in (no error)"=w459, "Find Fiducials"=w463, "Gluing Procedure in"=w466) -> ("error out"=w455:errorcluster, "Gluing Procedure out"=w457:refnum<class "Gluing Procedure.lvclass">)  [unwired: 7 in]
      n176 = call "Image Dispose.vi"("Archive?"=TRUE, "error in"=w455, "Gluing Procedure in"=w457) -> ("error out"=w453:errorcluster, "Gluing Procedure out"=w454:refnum<class "Gluing Procedure.lvclass">)  [unwired: 7 in]
      n177 = call "Update Worktable Fid Positions.vi"("error in"=w453, "Gluing Procedure in"=w454) -> ("error out"=w452:errorcluster, "Gluing Procedure out"=w451:refnum<class "Gluing Procedure.lvclass">)  [unwired: 8 in]
      n178 = call "Read Worktable.vi"("error in"=w452, "Gluing Procedure in"=w451) -> ("error out"=w445:errorcluster, "WorkTable out"=w444:refnum<class "WorkTable Class.lvclass">, "Gluing Procedure out"=w462:refnum<class "Gluing Procedure.lvclass">)  [unwired: 7 in]
      n179 = call "Format Fiducial Data.vi"("Path Fiducials"=w443, "Procedure Type"=Worktable_Mode."Gluing", "error in"=w445, "Worktable"=w444, "Console Log in"=w441) -> ("error out"=w446:errorcluster, "Formatted Fiducial Data"=w449:string, "Console Log out"=w448:refnum<class "Console Log.lvclass">)  [unwired: 4 in]
      n180 = call "Add Line.vi"("error in"=w446, "String"=w449, "Console Log in"=w448) -> ("error out"=w447:errorcluster, "Console Log out"=w450:refnum<class "Console Log.lvclass">)  [unwired: 7 in]
      n181 = call "Write Review Fiducials.vi"("error in (no error)"=w447, "Review Fiducials"=T17 {"Has been run?"=TRUE}, "Gluing Procedure in"=w462) -> ("error out"=w458:errorcluster, "Gluing Procedure out"=w460:refnum<class "Gluing Procedure.lvclass">)  [unwired: 7 in]
    }
    frame True {
      # "True means Cancel was pressed"
    }
  }
  "Gluing Procedure out" <- w6
  "Console Log out" <- w7
  "Step canceled?" <- w10
  n182 = invoke class="VI" method="FP.Close"(reference=w15, error in=w4) -> (error out=→"error out":errorcluster)  [unwired: 1 in, 2 out]
